vi "Read Report Path.vi"(11 "Test Report.Default in":refnum<class "Test Report.Default.lvclass">) -> (2 "Report Path":path, 3 "Test Report.Default out":refnum<class "Test Report.Default.lvclass">)   [LabVIEW 2013, in "Caraya.lvlib" / "Test Report.Default.lvclass"]
uses:
  Test Report.Default.lvclass
  Test Report.Default.lvclass/Test Report.Default.ctl
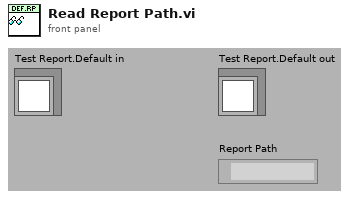
[diagram p1: front panel]
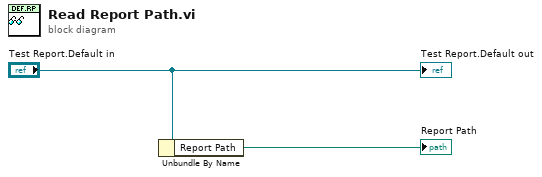
[diagram p0: block diagram]
diagram:
  n1 = Unbundle By Name("Test Report.Default in") -> ("Report Path"=→"Report Path":path)
  "Test Report.Default out" <- "Test Report.Default in"
